vi "cook.vi"(8 "error in (no error)":errorcluster, 11 "OrderPizza in":refnum<class "OrderPizza.lvclass">) -> (0 "error out":errorcluster, 3 "OrderPizza out":refnum<class "OrderPizza.lvclass">)   [LabVIEW 2010, in "CookBehaviors.lvlib" / "OrderPizza.lvclass"]
uses:
  OrderPizza.lvclass
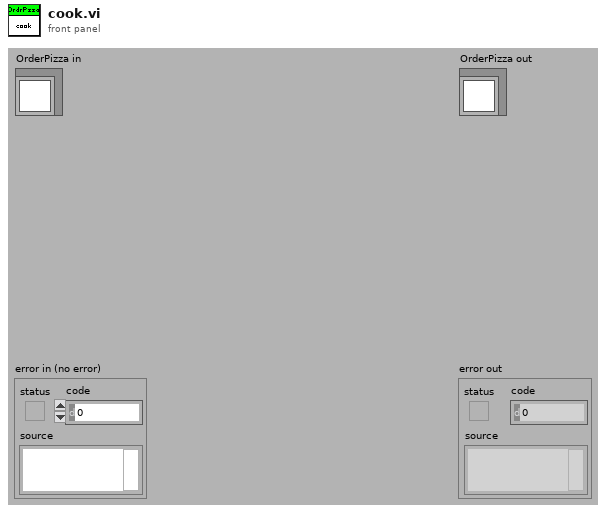
[diagram p1: front panel]
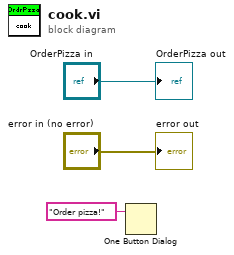
[diagram p0: block diagram]
diagram:
  n1 = One Button Dialog(message="Order pizza!") -> ()  [unwired: 1 in, 1 out]
  "error out" <- "error in (no error)"
  "OrderPizza out" <- "OrderPizza in"
